vi "GenerateChangedFilesList.vi"(6 "GUI Mode? {F)":bool, 7 "Output File Path":path=path "E:/sw-deps-monitor/changed-files.txt", 8 "error in (no error)":errorcluster, 9 "Branch 2":string="initial-ci-check-yml", 10 "Branch 1":string="main", 11 "Workspace Path":path=path "E:/sw-deps-monitor") -> (0 "error out":errorcluster)   [LabVIEW 2019, in "DepsWatch.lvlib"]
uses:
  DepsWatch.lvlib
  <vilib>/Hampel Software Engineering/Git API/Git API/GIT-api.lvclass/GIT-api.ctl
  <vilib>/Hampel Software Engineering/Git API/Git API/Accessors/GIT-Set Working Dir.vi
  <vilib>/Wiresmith Technology/G CLI/CLI Class/CLI.lvclass
  <vilib>/Hampel Software Engineering/Git API/Git API/GIT-api.lvclass
panel:
  out "std out":string
  in  "Tab Control":T1(tab)
  out "Args":string[](array[string])=["E:\\sw-deps-monitor", "main", "initial-ci-check-yml", "E:\\sw-deps-monitor\\changed-files.txt"]
  # "When in GUI Mode, the controls will be used, \nin CLI Mode the Args will be used"
  # "Workspace Path"
  # "Branch 1"
  # "Branch 2"
  # "Output File Path"
  # "Command to run the VI from terminal\n\ng-cli -v --lv-ver 2023 --arch 32 \"E:\\sw-deps-monitor\\CICD\\Reusables\\GenerateChangedFilesList.vi\" \n-- \"E:\\sw-deps-monitor\" \"main\" \"initial-ci-check-yml\" \"E:\\sw-deps-monitor\\changed-files.txt\""
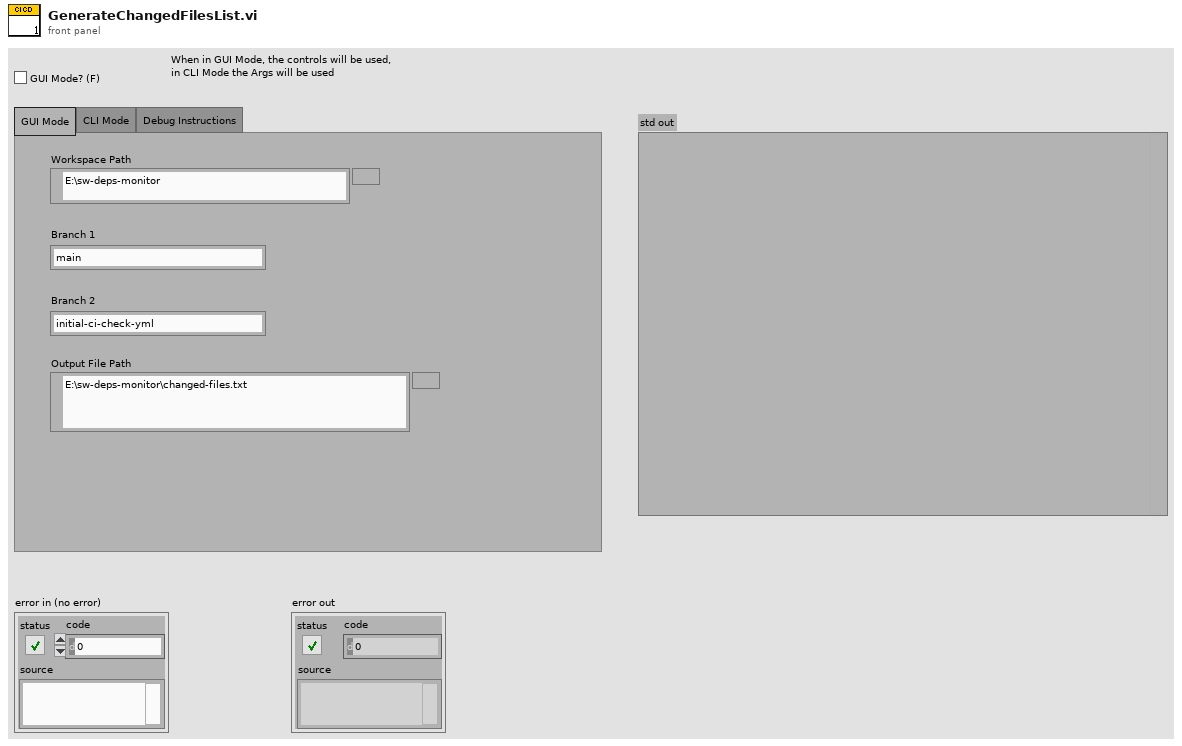
[diagram p1: front panel]
types:
  T1 = enum32{"GUI Mode", "CLI Mode", "Debug Instructions"}
  T2 = enum16{"open", "replace", "create", "open or create", "replace or create", "replace or create with confirmation"}
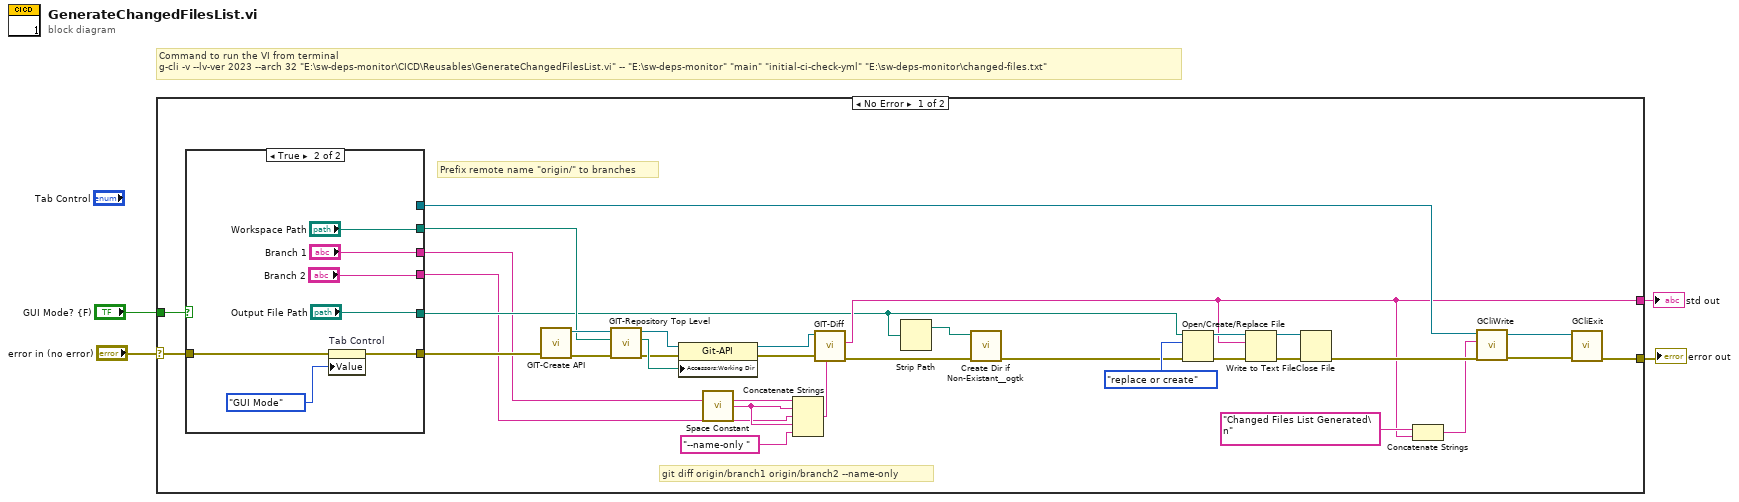
[diagram p0: block diagram]
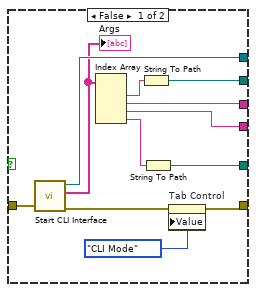
[diagram p2: hidden frame]
diagram:
  # "Command to run the VI from terminal\ng-cli -v --lv-ver 2023 --arch 32 \"E:\\sw-deps-monitor\\CICD\\Reusables\\GenerateChangedFilesList.vi\" -- \"E:\\sw-deps-monitor\" \"main\" \"initial-ci-check-yml\" \"E:\\sw-deps-monitor\\changed-files.txt\""
  n1 = case shown="No Error" "error in (no error)" {
    selector: "error in (no error)" -> [w27 w57]
    tunnel: "GUI Mode? {F)" -> [w28 _]
    tunnel: [w12 _] -> w2
    tunnel: [w15 w57] -> w1
    frame No Error {
      # "git diff origin/branch1 origin/branch2 --name-only"
      # "Prefix remote name \"origin/\" to branches"
      n2 = case shown="True" w28 {
        tunnel: [w48 "Branch 1"] -> w5
        tunnel: [w45 "Workspace Path"] -> w25
        tunnel: [w44 "Output File Path"] -> w10
        tunnel: [w47 "Branch 2"] -> w6
        tunnel: w27 -> [w43 w52]
        tunnel: [w41 w50] -> w26
        tunnel: [w42 _] -> w17
        frame False {
          n3 = call <vilib>:"Start CLI Interface.vi"("error in (no error)"=w43) -> ("error out"=w39:errorcluster, "Custom Parameters"=w38:string[], "CLI out"=w42:refnum<class "CLI.lvclass">)  [unwired: 7 in, 1 out]
          "Args" <- w38
          n4 = Index Array(array=w38) -> (element #1=w49:string, element #2=w48:string, element #3=w47:string, element #4=w46:string)  [unwired: 4 in]
          n5 = String To Path(string=w49) -> (path=w45:path)
          n6 = String To Path(string=w46) -> (path=w44:path)
          n7 = property on="Tab Control" class="TabCtl (strict)"(error in=w39, "Value"=enum32{"GUI Mode", "CLI Mode"}."CLI Mode" ("Tab Control")) -> (error out=w41:errorcluster)  [unwired: 1 in, 1 out]
        }
        frame True {
          n8 = property on="Tab Control" class="TabCtl (strict)"(error in=w52, "Value"=enum32{"GUI Mode", "CLI Mode"}."GUI Mode" ("Tab Control")) -> (error out=w50:errorcluster)  [unwired: 1 in, 1 out]
        }
      }
      n9 = call <vilib>:"GIT-Create API.vi"("error in"=w26) -> ("error out"=w33:errorcluster, "git-api out"=w36:refnum<class "GIT-api.lvclass">)  [unwired: 9 in]
      n10 = call <vilib>:"GIT-Repository Top Level.vi"("error in"=w33, "Current Path"=w25, "git-api in"=w36) -> ("error out"=w34:errorcluster, "Repo Top Level Path"=w35:path, "git-api out"=w37:refnum<class "GIT-api.lvclass">)  [unwired: 6 in]
      n11 = property class="Git-API"(reference=w37, error in=w34, "Accessors:Working Dir"=w35) -> (reference out=w31:refnum<class "GIT-api.lvclass">, error out=w32:errorcluster)
      n12 = call <vilib>:"Space Constant.vi"() -> ("String"=w24:string)
      n13 = Concatenate Strings(w5, w24, w6, w24, "--name-only " ("string")) -> (w30:string)
      n14 = call <vilib>:"GIT-Diff.vi"("param"=w30, "error in"=w32, "git-api in"=w31) -> ("error out"=w8:errorcluster, "std out"=w12:string)  [unwired: 6 in, 1 out]
      n15 = Strip Path(path=w10) -> (stripped path=w7:path)  [unwired: 1 out]
      n16 = call <userlib>:"Create Dir if Non-Existant__ogtk.vi"("error in (no error)"=w8, "Directory Path"=w7) -> ("error out"=w9:errorcluster)  [unwired: 7 in, 2 out]
      n17 = Open/Create/Replace File(file path (use dialog)=w10, error in=w9, operation (0:open)=T2."replace or create") -> (refnum out=w21:refnum<file>, error out=w22:errorcluster)  [unwired: 3 in, 1 out]
      n18 = Write to Text File(file (use dialog)=w21, text=w12, error in=w22) -> (refnum out=w19:refnum<file>, error out=w20:errorcluster)  [unwired: 1 in, 1 out]
      n19 = Close File(refnum=w19, error in=w20) -> (error out=w18:errorcluster)  [unwired: 1 out]
      n20 = Concatenate Strings("Changed Files List Generated\n" ("Text to Write"), w12) -> (w11:string)
      n21 = call "GCliWrite.vi"("error in (no error)"=w18, "Text to Write"=w11, "CLI in"=w17) -> ("error out"=w16:errorcluster, "CLI out"=w14:refnum<class "CLI.lvclass">)  [unwired: 7 in]
      n22 = call "GCliExit.vi"("error in (no error)"=w16, "CLI in"=w14) -> ("error out"=w15:errorcluster)  [unwired: 9 in]
    }
    frame Error {
    }
  }
  "error out" <- w1
  "std out" <- w2
